vi "LSX Get Hdi Keys.vi"(0 "lLSID":i32, 1 "plKey4":i32, 5 "plKey1":i32, 7 "plKey2":i32, 9 "plKey3":i32, 11 "error in (no error)":errorcluster) -> (3 "plKey4 out":i32, 4 "function return":i32, 6 "plKey1 out":i32, 8 "plKey2 out":i32, 10 "plKey3 out":i32, 15 "error out":errorcluster)   [LabVIEW 2018, in "Tango.lvlib"]
doc: "TANGOAPI int TANGOCALL LSX_GetHdiKeys (int lLSID, int *plKey1, int *plKey2, int *plKey3, int *plKey4);"
uses:
  <userlib>/Tango/Tango.lvlib
  <userlib>/Tango/Tango_DLL.dll
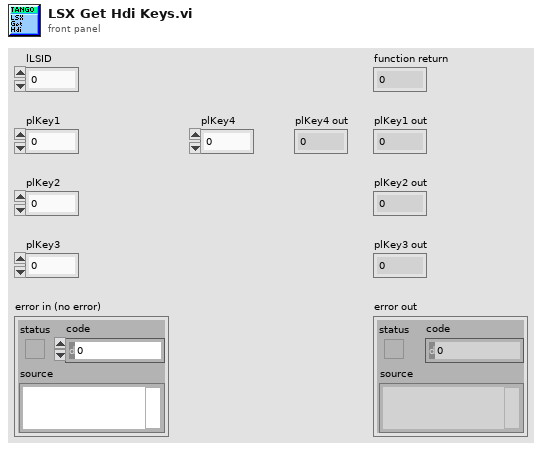
[diagram p1: front panel]
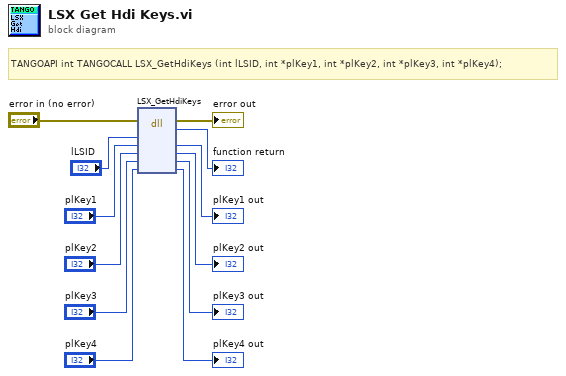
[diagram p0: block diagram]
diagram:
  # "TANGOAPI int TANGOCALL LSX_GetHdiKeys (int lLSID, int *plKey1, int *plKey2, int *plKey3, int *plKey4);"
  n1 = dll-call lib="C:/Program Files (x86)/National Instruments/LabVIEW 2018/user.lib/Tango/Tango_DLL.*" fn="LSX_GetHdiKeys"(error in="error in (no error)", "lLSID"="lLSID", "plKey1"="plKey1", "plKey2"="plKey2", "plKey3"="plKey3", "plKey4"="plKey4") -> (error out=→"error out":errorcluster, →"function return":i32, "plKey1"=→"plKey1 out":i32, "plKey2"=→"plKey2 out":i32, "plKey3"=→"plKey3 out":i32, "plKey4"=→"plKey4 out":i32)  [unwired: 3 in, 1 out]
